vi "QuickDrop Process Drop Information.vi"(0 "Listbox Contents":string[](array[string]), 1 "Project Item Refs":refnum<vi>[](array[refnum]), 2 "Project Items":string[](array[string]), 3 "App Refnum":refnum<vi>, 5 "Shortcut Info":string[][](array[string]), 7 "Text.Text":string, 9 "Shortcuts":string[](array[string]), 12 "Run for Plugin?":bool) -> (4 "Project VI Path":path, 6 "Palette Object Name":string)   [LabVIEW 2024]
uses:
  QD Suggestion.ctl
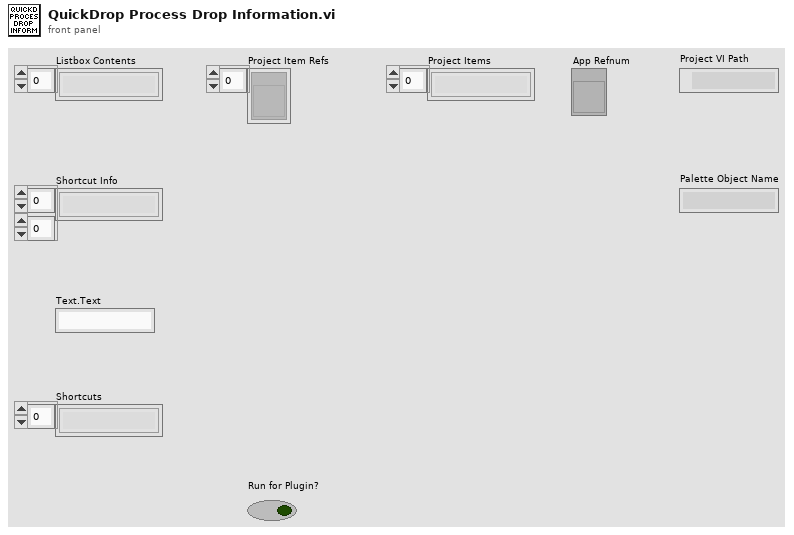
[diagram p1: front panel]
types:
  T1 = typedef "QD Suggestion.ctl" = cluster{"Data":string, "qd":string[], "Type":string}
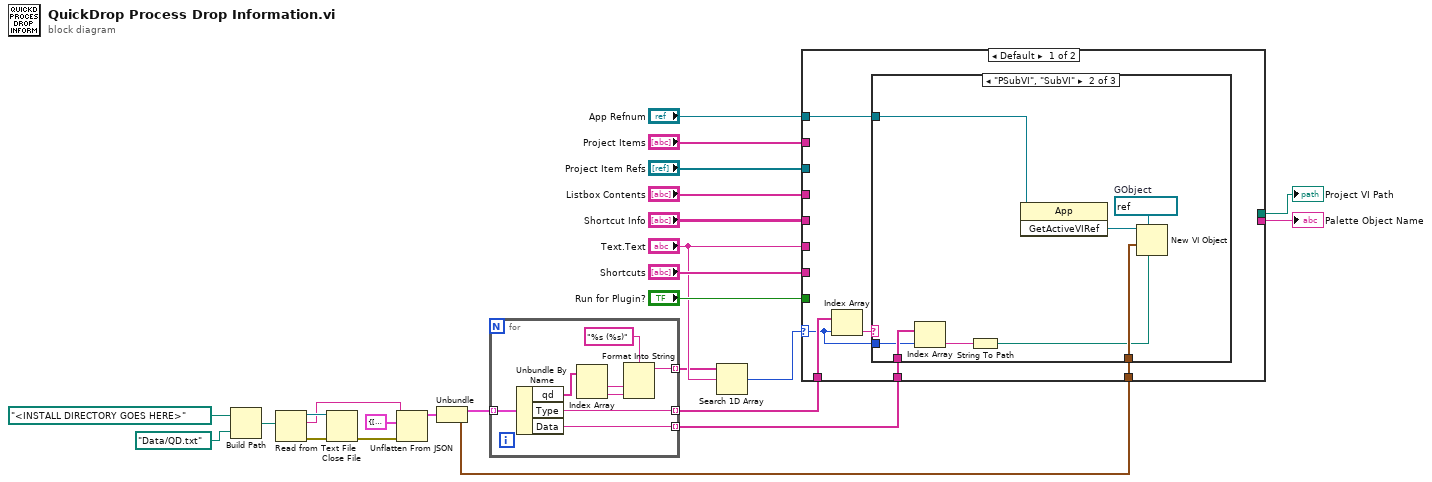
[diagram p0: block diagram]
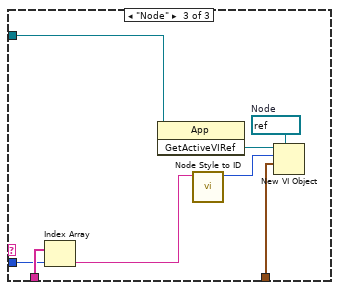
[diagram p3: hidden frame]
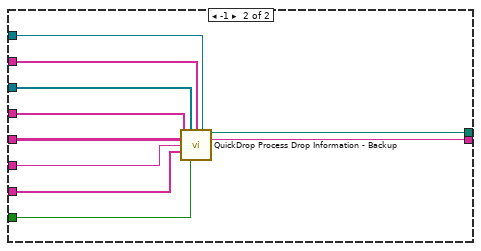
[diagram p4: hidden frame]
diagram:
  n1 = Build Path(base path=path "<INSTALL DIRECTORY GOES HERE>", name or relative path=path "Data/QD.txt" ("file (use dialog)")) -> (appended path=w1:path)
  n2 = Read from Text File(file (use dialog)=w1) -> (refnum out=w16:refnum<file>, text=w4:string, error out=w15:errorcluster)  [unwired: 3 in, 1 out]
  n3 = Close File(refnum=w16, error in=w15) -> (error out=w14:errorcluster)  [unwired: 1 out]
  n4 = Unflatten From JSON(JSON string=w4, type and defaults=cluster{T1[], cluster{"Left":i32, "Top":i32}} {[], {"Left"=0, "Top"=0}} ("cluster"), error in (no error)=w14) -> (value=w12:cluster{T1[], cluster{"Left":i32, "Top":i32}})  [unwired: 4 in, 1 out]
  n5 = Unbundle(w12) -> (w11:T1[], w10:cluster{"Left":i32, "Top":i32})
  n6 = for {
    tunnel: w11 -> [w33] mode=indexing
    tunnel: [w28] -> w5 mode=indexing
    tunnel: [w27] -> w9 mode=indexing
    tunnel: [w26] -> w8 mode=indexing
    n7 = Unbundle By Name(w33) -> ("qd"=w31:string[], "Type"=w26:string, "Data"=w27:string)
    n8 = Index Array(array=w31) -> (element #1=w30:string, element #2=w29:string)  [unwired: 2 in]
    n9 = Format Into String(format string="%s (%s)", w30, w29) -> (resulting string=w28:string)  [unwired: 2 in, 1 out]
  }
  n10 = Search 1D Array(1D array=w5, element="Text.Text") -> (index of element=w7:i32)  [unwired: 1 in]
  n11 = case shown="Default" w7 {
    selector: w7 -> [w35 _]
    tunnel: "Run for Plugin?" -> [_ w65]
    tunnel: "Project Item Refs" -> [_ w64]
    tunnel: "Project Items" -> [_ w63]
    tunnel: "Listbox Contents" -> [_ w62]
    tunnel: "Shortcuts" -> [_ w61]
    tunnel: "Shortcut Info" -> [_ w60]
    tunnel: [_ w59] -> w19
    tunnel: [_ w58] -> w18
    tunnel: "App Refnum" -> [w36 w57]
    tunnel: "Text.Text" -> [_ w56]
    tunnel: w10 -> [w37 _]
    tunnel: w9 -> [w34 _]
    tunnel: w8 -> [w39 _]
    frame Default {
      n12 = Index Array(array=w39, index=w35) -> (element=w38:string)
      n13 = case shown="\"PSubVI\", \"SubVI\"" w38 {
        tunnel: w37 -> [_ w45 w53]
        tunnel: w36 -> [_ w44 w52]
        tunnel: w35 -> [_ w41 w49]
        tunnel: w34 -> [_ w42 w50]
        frame Default {
        }
        frame "PSubVI", "SubVI" {
          w46 = refnum<vi> refnum  # GObject
          n14 = Index Array(array=w42, index=w41) -> (element=w40:string)
          n15 = String To Path(string=w40) -> (path=w43:path)
          n16 = invoke class="App" method="GetActiveVIRef"(reference=w44) -> ("GetActiveVIRef"=w47:refnum<vi>)  [unwired: 2 in, 2 out]
          n17 = New VI Object(vi object class=w46, owner refnum=w47, position/next to=w45, 6:w43) -> ()  [unwired: 4 in, 2 out]
        }
        frame "Node" {
          w54 = refnum<vi> refnum  # Node
          n18 = Index Array(array=w50, index=w49) -> (element=w48:string)
          n19 = invoke class="App" method="GetActiveVIRef"(reference=w52) -> ("GetActiveVIRef"=w55:refnum<vi>)  [unwired: 2 in, 2 out]
          n20 = call "Node Style to ID.vi"("Function Name"=w48) -> ("Function ID"=w51:i32)  [unwired: 9 in, 1 out]
          n21 = New VI Object(vi object class=w54, owner refnum=w55, style=w51, position/next to=w53) -> ()  [unwired: 4 in, 2 out]
        }
      }
    }
    frame -1 {
      n22 = call <resource>:"QuickDrop Process Drop Information - Backup.vi"("Listbox Contents"=w62, "Project Item Refs"=w64, "Project Items"=w63, "App Refnum"=w57, "Shortcut Info"=w60, "Text.Text"=w56, "Shortcuts"=w61, "Run for Plugin?"=w65) -> ("Project VI Path"=w58:path, "Palette Object Name"=w59:string)  [unwired: 6 in]
    }
  }
  "Project VI Path" <- w18
  "Palette Object Name" <- w19
